vi "Add Tx Generic Command Section.vi"(8 "error in":errorcluster, 11 "Tx generic ref in":T1 format="%.0x") -> (0 "error out":errorcluster, 2 "Tx generic command section ref out":T1 format="%.0x", 3 "Tx generic ref out":T1 format="%.0x")   [LabVIEW 2020, in "AIM ARINC 664 Scripting.lvlib"]
uses:
  AIM ARINC 664 Scripting.lvlib
  <vilib>/NI VeriStand/Custom Device API/Custom Device Item Ref.ctl
  Constants.vi
  <vilib>/NI VeriStand/Custom Device API/Custom Device API.lvlib
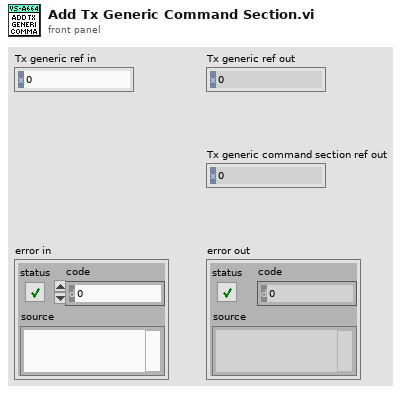
[diagram p1: front panel]
types:
  T1 = typedef "Custom Device API.lvlib/Custom Device Item Ref.ctl" = u64
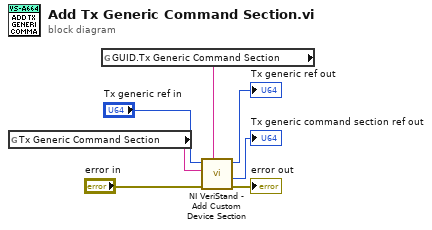
[diagram p0: block diagram]
diagram:
  n1 = global read "Constants.vi" "Tx Generic Command Section"() -> (w4:string)
  n2 = global read "Constants.vi" "GUID.Tx Generic Command Section"() -> (w6:string)
  n3 = call <vilib>:"NI VeriStand - Add Custom Device Section.vi"("GUID (Default Section)"=w6, "error in (no error)"="error in", "Section Name"=w4, "Parent Ref in"="Tx generic ref in") -> ("error out"=→"error out":errorcluster, "Section Ptr"=→"Tx generic command section ref out":T1, "Parent Ref out"=→"Tx generic ref out":T1)  [unwired: 4 in, 1 out]
